vi "19572 Series STOP.vi"(8 "error in (no error)":errorcluster, 11 "VISA resource in":refnum<visa-resource-name>) -> (0 "error out":errorcluster, 3 "VISA resource out":refnum<visa-resource-name>)   [LabVIEW 2015]
panel:
  out "output command":string
  # "STOP"
  # "This is valid for both:\n19572 & 19052"
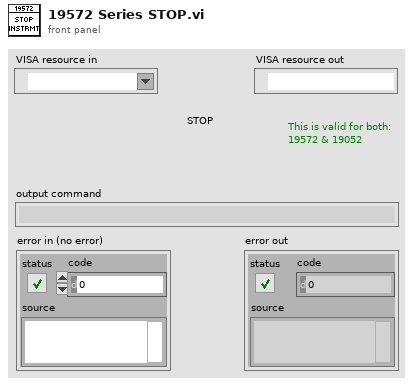
[diagram p1: front panel]
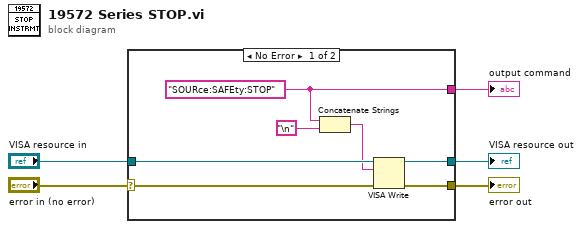
[diagram p0: block diagram]
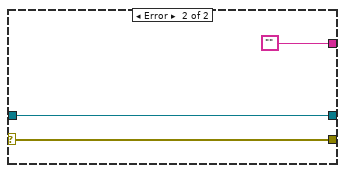
[diagram p2: hidden frame]
diagram:
  n1 = case shown="No Error" "error in (no error)" {
    selector: "error in (no error)" -> [w11 w15]
    tunnel: [w12 w15] -> w5
    tunnel: "VISA resource in" -> [w9 w14]
    tunnel: [w8 w14] -> w2
    tunnel: [w7 ""] -> w1
    frame No Error {
      w7 = "SOURce:SAFEty:STOP"
      n2 = Concatenate Strings(w7, "\n") -> (w6:string)
      n3 = VISA Write(VISA resource name=w9, write buffer=w6, error in (no error)=w11) -> (VISA resource name out=w8:refnum<visa-resource-name>, error out=w12:errorcluster)  [unwired: 1 out]
    }
    frame Error {
    }
  }
  "error out" <- w5
  "VISA resource out" <- w2
  "output command" <- w1
